vi "DriveForward2.vi"   [LabVIEW 2015]
uses:
  ShiftGlobals.vi
  RobotCode/TwoBallAutoGlobals.vi
types:
  T1 = typedef "WPI_MotorControlDeviceRef.ctl" = cluster{"DeviceStatus":errorcluster, "Type":T2, "PWM":cluster{"PWM Channel":T3, "DeadBand":T4}, "CAN":cluster{"Device Number":u8, "Control Mode":T5, "Semaphore":T6, "Max Vout":dbl, "TalonSRX Control Mode":T7}, "Invert":bool}
  T2 = typedef "WPI_MotorControlType.ctl" = enum16{"PWM", "CAN", "CANTalonSRX"}
  T3 = typedef "FPGA_DIOPWMChannel.ctl" = enum8{"PWM 0", "PWM 1", "PWM 2", "PWM 3", "PWM 4", "PWM 5", "PWM 6", "PWM 7", "PWM 8", "PWM 9", "PWM MXP 0", "PWM MXP 1", "PWM MXP 2", "PWM MXP 3", "PWM MXP 4", "PWM MXP 5", "PWM MXP 6", "PWM MXP 7", "PWM MXP 8", "PWM MXP 9", "Invalid"}
  T4 = typedef "WPI_PWMDeadband.ctl" = cluster{"Name":string, "maxPositivePwm":i32, "minPositivePwm":i32, "centerPwm":i32, "maxNegativePwm":i32, "minNegativePwm":i32, "angularRange":u16}
  T5 = typedef "WPI_CANJaguar_ControlMode.ctl" = enum8{"Percent VBus", "Current", "Speed", "Position", "Voltage"}
  T6 = typedef "Semaphore RefNum" = refnum<k1>
  T7 = typedef "WPI_CANTalonSRX_APIControlMode.ctl" = enum8{"Percent VBus", "Speed", "Position", "Slave", "Unchanged / Invalid", "Voltage Compensation", "Current", "Motion Profile"}
  T8 = typedef "WPI_CANTalonSRX_GlobalStatus.ctl" = cluster{"Applied Throttle":dbl, "Module Enabled":bool, "CAN Error":errorcluster, "Closed Loop Error":dbl, "Forward Limit Switch Closed":bool, "Reverse Limit Switch Closed":bool, "Sensor Position":dbl, "Sensor Velocity":dbl, "Current":dbl, "Sticky Fault - Over Temp":bool, "Sticky Fault - Under Voltage":bool, "Sticky Fault - Forward Limit":bool, "Sticky Fault - Reverse Limit":bool, "Sticky Fault - Forward Soft Limit":bool, "Sticky Fault - Reverse Soft Limit":bool, "Brake is Enabled":bool, "Encoder Position":dbl, "Encoder Velocity":dbl, "Encoder Index Count":dbl, "Encoder A Pin State":bool, "Encoder B Pin State":bool, "Encoder Index Pin State":bool, "Analog In":dbl, "Analog In Velocity":dbl, "Temperature (C)":dbl, "Battery Voltage":dbl, "Control 5 Is Supported":bool, "Current Profile Slot Select":dbl, "Pos Div 8":bool, "Vel Div 4":bool, "Pulse Width Position":i32, "Pulse Width Velocity":i32, "Pulse Width Rise To Rise (us)":i32, "Pulse Width Rise To Fall (us)":i32, "Mot Prof Active Is Under Run":bool, "Mot Prof Active Has Under Run":bool, "Mot Prof Active Is Last":bool, "Mot Prof Active Velocity Only":bool, "Mot Prof Active Is Valid":bool, "Mot Prof Buffer Is Full":bool, "Mot Prof Active Profile Slot Select":i32, "Mot Prof NextID":i32, "Mot Prof Count":i32, "Mot Prof Active Velocity":dbl, "Mot Prof Active Position":dbl, "Mot Prof Output Enable":i32}
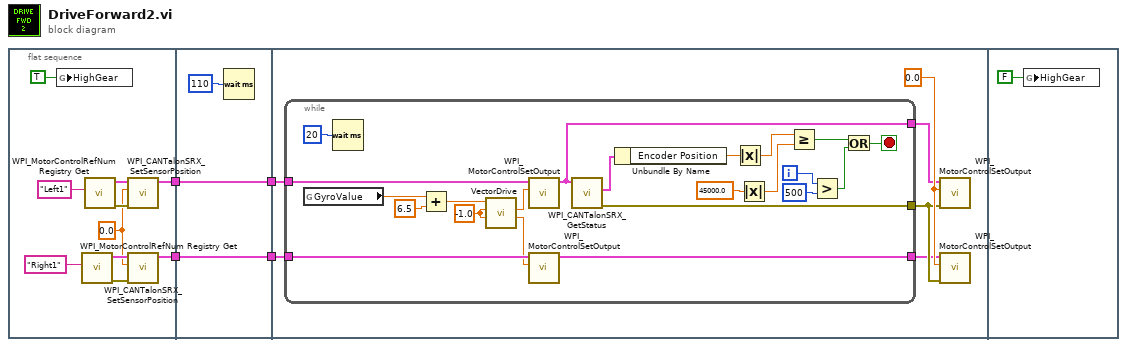
[diagram p0: block diagram]
diagram:
  n1 = flat-sequence {
    tunnel: [w7] -> w4
    tunnel: [w6] -> w3
    tunnel: w4 -> [w17]
    tunnel: [w17] -> w1
    tunnel: w3 -> [w16]
    tunnel: [w16] -> w2
    tunnel: w2 -> [w21]
    tunnel: w1 -> [w20]
    frame #0 {
      w8 = 0.0 ("New Sensor Position")
      n2 = global write "ShiftGlobals.vi" "HighGear"(TRUE ("HighGear")) -> ()
      n3 = call <vilib>:"WPI_MotorControlRefNum Registry Get.vi"("refnum name"="Right1") -> ("error out"=w12:errorcluster, "MotorControlDevRef"=w11:T1)  [unwired: 9 in]
      n4 = call <vilib>:"WPI_MotorControlRefNum Registry Get.vi"("refnum name"="Left1") -> ("error out"=w10:errorcluster, "MotorControlDevRef"=w9:T1)  [unwired: 9 in]
      n5 = call <vilib>:"WPI_CANTalonSRX_SetSensorPosition.vi"("error in (no error)"=w10, "New Sensor Position"=w8, "CAN Talon SRX Ref"=w9) -> ("CAN Talon SRX Ref"=w6:T1)  [unwired: 7 in, 1 out]
      n6 = call <vilib>:"WPI_CANTalonSRX_SetSensorPosition.vi"("error in (no error)"=w12, "New Sensor Position"=w8, "CAN Talon SRX Ref"=w11) -> ("CAN Talon SRX Ref"=w7:T1)  [unwired: 7 in, 1 out]
    }
    frame #1 {
      n7 = Wait (ms)(milliseconds to wait=u32 110) -> ()  [unwired: 1 out]
    }
    frame #2 {
      w23 = 0.0 ("Output")
      n8 = while {
        tunnel: [w34] -> w22
        tunnel: w21 -> [w33]
        tunnel: w20 -> [w32]
        tunnel: [w31] -> w19
        tunnel: [w30] -> w18
        i -> [w40]
        stop <- w42 stop-if-true
        w27 = -1.0 ("Output")
        n9 = global read "TwoBallAutoGlobals.vi" "GyroValue"() -> (w26:dbl)
        n10 = Wait (ms)(milliseconds to wait=u32 20) -> ()  [unwired: 1 out]
        n11 = Add(x=w26, y=6.5 ("setpoint")) -> (x+y=w24:dbl)
        n12 = call "VectorDrive.vi"("RightMotorInput"=w27, "LeftMotorInput"=w27, "setpoint"=w24) -> ("RightMotorOutput"=w28:dbl, "LeftMotorOutput"=w29:dbl)  [unwired: 7 in]
        n13 = call <vilib>:"WPI_MotorControlSetOutput.vi"("Output"=w29, "MotorControlDevRef"=w33) -> ("MotorControlDevRef"=w31:T1)  [unwired: 7 in, 2 out]
        n14 = call <vilib>:"WPI_MotorControlSetOutput.vi"("Output"=w28, "MotorControlDevRef"=w32) -> ("MotorControlDevRef"=w30:T1)  [unwired: 7 in, 2 out]
        n15 = call <vilib>:"WPI_CANTalonSRX_GetStatus.vi"("CAN Talon SRX Ref"=w31) -> ("error out"=w34:errorcluster, "Talon SRX Status"=w44:T8)  [unwired: 8 in, 1 out]
        n16 = Unbundle By Name(w44) -> ("Encoder Position"=w38:dbl)
        n17 = Absolute Value(x=w38) -> (abs(x)=w37:dbl)
        n18 = Absolute Value(x=45000.0) -> (abs(x)=w36:dbl)
        n19 = Greater Or Equal?(x=w37, y=w36) -> (x >= y?=w43:bool)
        n20 = Greater?(x=w40, y=500) -> (0:w41:bool)
        n21 = Or(x=w43, y=w41) -> (x .or. y?=w42:bool)
      }
      n22 = call <vilib>:"WPI_MotorControlSetOutput.vi"("error in (no error)"=w22, "Output"=w23, "MotorControlDevRef"=w19) -> ()  [unwired: 6 in, 3 out]
      n23 = call <vilib>:"WPI_MotorControlSetOutput.vi"("error in (no error)"=w22, "Output"=w23, "MotorControlDevRef"=w18) -> ()  [unwired: 6 in, 3 out]
    }
    frame #3 {
      n24 = global write "ShiftGlobals.vi" "HighGear"(FALSE ("HighGear")) -> ()
    }
  }
